vi "Fit VI window.vi"(8 "error in (no error)":errorcluster, 11 "VI Ref (calling VI)":refnum<vi>) -> (0 "error out":errorcluster)   [LabVIEW 2017]
panel:
  in  "border spacing (2 px)":i32=2
  out "dup VI Ref":refnum<vi>
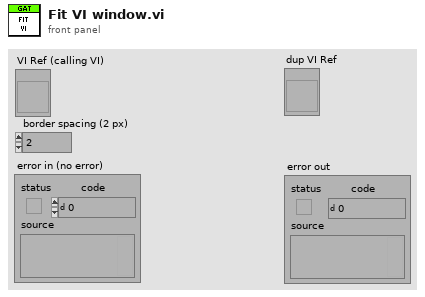
[diagram p1: front panel]
types:
  T1 = typedef "LVRectTypeDef.ctl" = cluster{"Left":i16, "Top":i16, "Right":i16, "Bottom":i16}
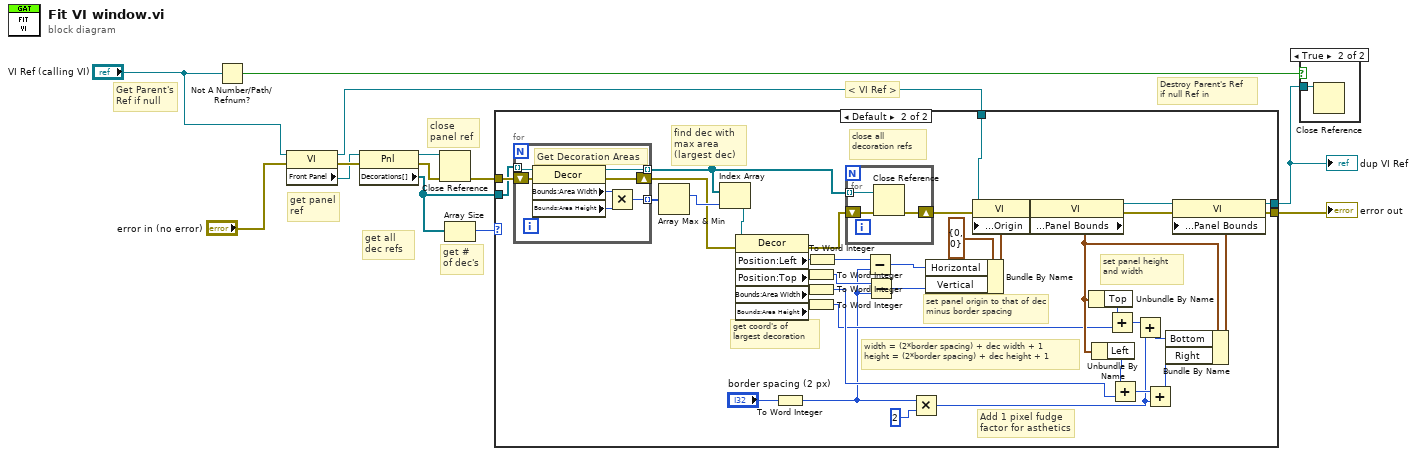
[diagram p0: block diagram]
diagram:
  # "Destroy Parent's Ref\nif null Ref in"
  # "Get Parent's\nRef if null"
  # "get # of dec's"
  # "get panel ref"
  # "get all dec refs"
  # "close panel ref"
  # "< VI Ref >"
  n1 = Not A Number/Path/Refnum?(number/path/refnum="VI Ref (calling VI)") -> (NaN/Path/Refnum?=w3:bool)
  n2 = property on="Property Node" class="VI"(reference="VI Ref (calling VI)", error in="error in (no error)") -> (reference out=w13:refnum<vi>, error out=w11:errorcluster, "Front Panel"=w8:refnum<vi>)
  n3 = property on="Property Node" class="Pnl"(reference=w8, error in=w11) -> (reference out=w12:refnum<vi>, error out=w10:errorcluster, "Decorations[]"=w5:refnum<vi>[])
  n4 = Close Reference(reference=w12, error in (no error)=w10) -> (error out=w7:errorcluster)
  n5 = Array Size(array=w5) -> (size(s)=w4:i32)
  n6 = case shown="Default" w4 {
    tunnel: w13 -> [w15 w53]
    tunnel: w7 -> [w14 w36]
    tunnel: [w14 w24] -> w6
    tunnel: [w15 w23] -> w2
    tunnel: w5 -> [_ w22]
    frame 0 {
      # "do nothing if no decorations"
    }
    frame Default {
      # "width = (2*border spacing) + dec width + 1\nheight = (2*border spacing) + dec height + 1"
      # "set panel height and width"
      # "set panel origin to that of dec minus border spacing"
      # "close all  decoration refs"
      # "get coord's of largest decoration"
      # "Add 1 pixel fudge factor for asthetics"
      # "find dec with max area (largest dec)"
      n7 = for {
        tunnel: w22 -> [w62] mode=indexing
        tunnel: [w59] -> w35 mode=indexing
        shift-right: [w57] -> w31
        shift-left: w36 -> [w58]
        tunnel: [w56] -> w33 mode=indexing
        # "Get Decoration Areas"
        n8 = property class="Decor"(reference=w62, error in=w58) -> (reference out=w56:refnum<vi>, error out=w57:errorcluster, "Bounds:Area Width"=w61:u32, "Bounds:Area Height"=w60:u32)
        n9 = Multiply(x=w61, y=w60) -> (x*y=w59:u32)
      }
      n10 = Array Max & Min(array=w35) -> (max index (indices)=w34:i32)  [unwired: 3 out]
      n11 = Index Array(array=w33, index=w34) -> (element=w32:refnum<vi>)
      n12 = property class="Decor"(reference=w32, error in=w31) -> (error out=w30:errorcluster, "Position:Left"=w39:i32, "Position:Top"=w42:i32, "Bounds:Area Width"=w47:u32, "Bounds:Area Height"=w45:u32)  [unwired: 1 out]
      n13 = To Word Integer(number="border spacing (2 px)") -> (16bit integer=w16:i16)
      n14 = To Word Integer(number=w42) -> (16bit integer=w17:i16)
      n15 = To Word Integer(number=w47) -> (16bit integer=w20:i16)
      n16 = To Word Integer(number=w45) -> (16bit integer=w19:i16)
      n17 = To Word Integer(number=w39) -> (16bit integer=w18:i16)
      n18 = for {
        tunnel: w33 -> [w65] mode=indexing
        shift-right: [w63] -> w27
        shift-left: w30 -> [w64]
        n19 = Close Reference(reference=w65, error in (no error)=w64) -> (error out=w63:errorcluster)
      }
      n20 = Subtract(x=w18, y=w16) -> (x-y=w40:i16)
      n21 = Subtract(x=w17, y=w16) -> (x-y=w41:i16)
      n22 = Multiply(x=w16, y=i16 2) -> (x*y=w21:i16)
      n23 = Bundle By Name(cluster=cluster{"Horizontal":i16, "Vertical":i16} {"Horizontal"=0, "Vertical"=0} ("Front Panel Window:Origin"), "Horizontal"=w40, "Vertical"=w41) -> (w37:cluster{"Horizontal":i16, "Vertical":i16})
      n24 = property on="Property Node" class="VI"(reference=w53, error in=w27, "Front Panel Window:Origin"=w37) -> (reference out=w54:refnum<vi>, error out=w26:errorcluster)
      n25 = property on="Property Node" class="VI"(reference=w54, error in=w26) -> (reference out=w55:refnum<vi>, error out=w25:errorcluster, "Front Panel Window:Panel Bounds"=w43:T1)
      n26 = Unbundle By Name(w43) -> ("Top"=w44:i16)
      n27 = Unbundle By Name(w43) -> ("Left"=w46:i16)
      n28 = Add(x=w44, y=w19) -> (x+y=w51:i16)
      n29 = Add(x=w46, y=w20) -> (x+y=w49:i16)
      n30 = Add(x=w51, y=w21) -> (x+y=w52:i16)
      n31 = Add(x=w49, y=w21) -> (x+y=w50:i16)
      n32 = Bundle By Name(cluster=w43, "Bottom"=w52, "Right"=w50) -> (w48:T1)
      n33 = property on="Property Node" class="VI"(reference=w55, error in=w25, "Front Panel Window:Panel Bounds"=w48) -> (reference out=w23:refnum<vi>, error out=w24:errorcluster)
    }
  }
  "error out" <- w6
  "dup VI Ref" <- w2
  n34 = case shown="True" w3 {
    tunnel: w2 -> [_ w66]
    frame False {
    }
    frame True {
      n35 = Close Reference(reference=w66) -> ()  [unwired: 1 in, 1 out]
    }
  }
